vi "Fast ABR.vi"(11 "State (in)":T19) -> (3 "State (out)":T19)   [LabVIEW 2020]
uses:
  epl-vi-lib/Utility VIs/Buttons/KCheckmarkBoolean 2.ctl
  CFTS SubVIs/CFTS-Experiment State.ctl
  Typedefs/FABR-Analysis State.ctl
  <vilib>/printing/EasyPrintingControls.llb/layout_options.ctl
  <vilib>/printing/EasyPrintingControls.llb/orientation.ctl
  <vilib>/printing/EasyPrintingControls.llb/panel_scaling_for_page.ctl
  <vilib>/printing/EasyPrintingControls.llb/margins.ctl
  <vilib>/printing/EasyPrintingControls.llb/margin_values.ctl
  <vilib>/printing/EasyPrintingControls.llb/measurement_system.ctl
  <vilib>/printing/EasyPrintingControls.llb/printer_options.ctl
  <vilib>/printing/EasyPrintingControls.llb/printing_method.ctl
  <vilib>/printing/EasyPrintingControls.llb/color_or_monochrome.ctl
  <vilib>/printing/EasyPrintingControls.llb/page_header_options.ctl
  <vilib>/printing/EasyPrintingControls.llb/page_headers.ctl
  <vilib>/printing/EasyPrintingControls.llb/page_header_content_options.ctl
  Typedefs/FABR-Parameters/FABR-Parameters.xctl
  Typedefs/FABR-Status.ctl
  Typedefs/FABR-Queue Data.ctl
  Typedefs/FABR-Parameters.ctl
  Typedefs/FABR-Stimulus.ctl
  Typedefs/FABR-Sequence.ctl
  Typedefs/FABR-Order.ctl
  Typedefs/FABR-Response.ctl
  Threshold Estimation VIs/ABR3-Threshold Estimation Parameters.ctl
  Typedefs/FABR-Stimulus Condition.ctl
  epl-vi-lib/PXI DAQ VIs/AIDI/Typedefs/AIDI-Action.ctl
  CFTS SubVIs/CFTS-Options.ctl
  <vilib>/printing/EasyPrintingControls.llb/contents.ctl
  931a586e-3910-4d06-be6a-8dff1fbf7332.vi
  epl-vi-lib/Utility VIs/Math VIs/LinSpace (start-stop-step).vi
  epl-vi-lib/Utility VIs/File IO VIs/Read Write Anything/Read Anything.vi
  <vilib>/printing/EasyPrinting.llb/Easy Print VI Panel or Documentation (refnum).vi
  <vilib>/Utility/NIReport.llb/NI_ReportGenerationCore.lvlib
panel:
  in  "Params":T5(xcontrol)
  in  "Start":bool
  in  "Run":i32
  in  "Number":i32
  in  "ID":string
  in  "Stop":bool
  in  "layout options":T6={"orientation (unchanged)"=0, "panel scaling for page (unchanged)"=0, "margins"={"override VI margins (false)"=FALSE, "margins (1.00)"={"top"=1.0, "left"=1.0, "right"=1.0, "bottom"=1.0}, "measurement system (default)"=0}, "printer options"={"destination printer name (current)"="", "printing method (unchanged)"=0, "color or monochrome (unchanged)"=0}, "page header options"={"page headers (unchanged)"=0, "page header content options"={"Include VI Name"=TRUE, "Include VI Path"=TRUE, "Include Last Modification Date"=TRUE, "Include Date Printed"=TRUE, "Include Page Number"=TRUE, "Include VI Icon"=TRUE}}} {"page header options"."page headers (unchanged)" items=["Unchanged", "Include page headers", "Do not include page headers"]; "printer options"."color or monochrome (unchanged)" items=["Unchanged", "Color/grayscale", "Monochrome"]; "printer options"."printing method (unchanged)" items=["Unchanged", "Standard", "PostScript", "Bitmap"]; "panel scaling for page (unchanged)" items=["Unchanged", "No Scaling", "Scale front panel to fit"]; "orientation (unchanged)" items=["Unchanged", "portrait", "landscape"]; "margins"."measurement system (default)" items=["Default", "US", "Metric"]; "margins"."margins (1.00)"."right" format="%.2f"; "margins"."margins (1.00)"."bottom" format="%.2f"; "margins"."margins (1.00)"."top" format="%.2f"; "margins"."margins (1.00)"."left" format="%.2f"}
  in  "NOTES":string
  in  "Scale":dbl=1.0 min=1.0 max=5.0 step=0.5
  out "Frej":dbl(slide) scale=0.0..1.0
  in  "RejThr":dbl caption="Reject at (uV)"
  in  "Override":bool
  in  "AvsF Axis":dbl(slide) caption="Frequency (kHz)" min=0.0 scale=0.0..3.0 scale format="%#.2g"
  out "Raw":dbl[](graph)
  out "AvsFLegend":i32(listbox)
  out "AvsF":cluster{dbl[], dbl[]}[](graph)
  out "IOLegend":i32(listbox)
  in  "YAxis":dbl(slide) caption="Level (dB SPL)" scale=0.0..13.5
  in  "XAxis":dbl(slide) caption="Frequency (kHz)" min=0.0 scale=0.0..4.0 scale format="%#.2g"
  out "Neural":cluster{dbl[], dbl[]}[](graph)
  out "Analysis":T18
  out "finished":errorcluster
  in  "Normalize traces":T20=TRUE caption="Normalize individual traces"
  out "I-O":cluster{dbl[], dbl[]}[](graph)
  # "Freq X Level X Time"
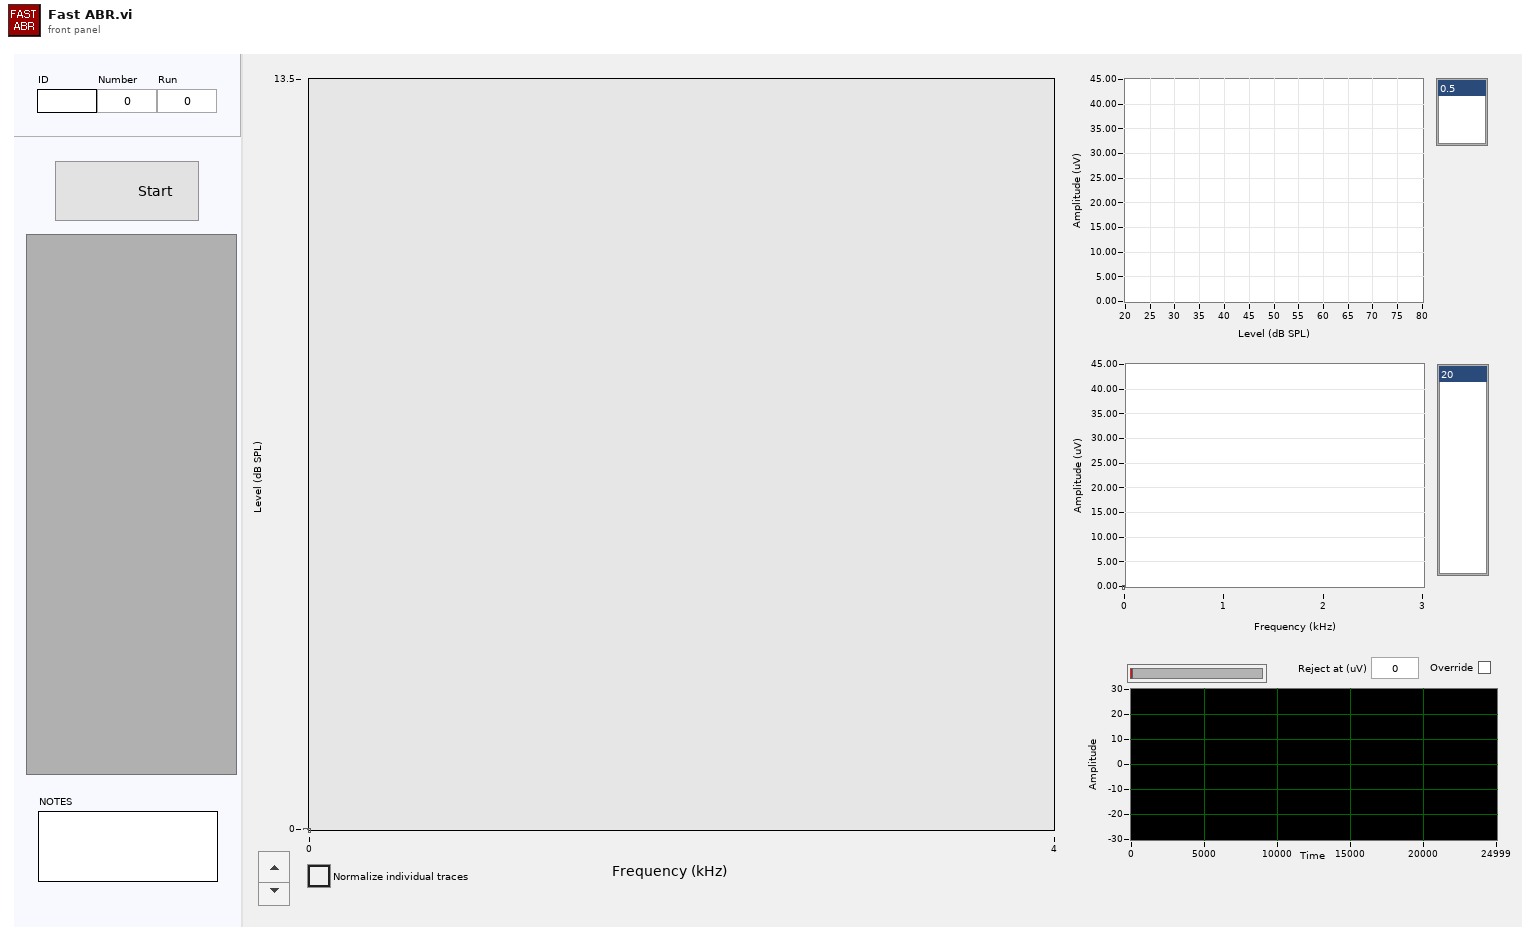
[diagram p1: front panel]
types:
  T1 = typedef "FABR-Stimulus.ctl" = cluster{"Destination":string, "Rep rate (/sec)":dbl, "Alternate Polarity":bool, "Duration (ms)":dbl, "Ramp (ms)":dbl, "Fs (Hz)":dbl, "Frame size (s)":dbl}
  T2 = typedef "FABR-Sequence.ctl" = cluster{"Freq":cluster{"Start (kHz)":dbl, "Stop (kHz)":dbl, "Step (oct)":dbl, "Skip (oct)":dbl}, "Level":cluster{"Start (dB)":i32, "Stop (dB)":i32, "Step (dB)":i32}, "Order":T3}
  T3 = typedef "FABR-Order.ctl" = enum16{"Interleaved"}
  T4 = typedef "FABR-Response.ctl" = cluster{"Gain":dbl, "Averages":i32, "Window (ms)":sgl, "Fs (Hz)":dbl, "Save raw":bool}
  T5 = cluster{"Stimulus":T1, "Sequence":T2, "Response":T4, "Reject":dbl}
  T6 = typedef "NI_ReportGenerationCore.lvlib/layout_options.ctl" = cluster{"orientation (unchanged)":T7, "panel scaling for page (unchanged)":T8, "margins":T9, "printer options":T12, "page header options":T15}
  T7 = typedef "NI_ReportGenerationCore.lvlib/orientation.ctl" = u16
  T8 = typedef "NI_ReportGenerationCore.lvlib/panel_scaling_for_page.ctl" = u16
  T9 = typedef "NI_ReportGenerationCore.lvlib/margins.ctl" = cluster{"override VI margins (false)":bool, "margins (1.00)":T10, "measurement system (default)":T11}
  T10 = typedef "NI_ReportGenerationCore.lvlib/margin_values.ctl" = cluster{"top":dbl, "left":dbl, "right":dbl, "bottom":dbl}
  T11 = typedef "NI_ReportGenerationCore.lvlib/measurement_system.ctl" = u16
  T12 = typedef "NI_ReportGenerationCore.lvlib/printer_options.ctl" = cluster{"destination printer name (current)":string, "printing method (unchanged)":T13, "color or monochrome (unchanged)":T14}
  T13 = typedef "NI_ReportGenerationCore.lvlib/printing_method.ctl" = u16
  T14 = typedef "NI_ReportGenerationCore.lvlib/color_or_monochrome.ctl" = u16
  T15 = typedef "NI_ReportGenerationCore.lvlib/page_header_options.ctl" = cluster{"page headers (unchanged)":T16, "page header content options":T17}
  T16 = typedef "NI_ReportGenerationCore.lvlib/page_headers.ctl" = u16
  T17 = typedef "NI_ReportGenerationCore.lvlib/page_header_content_options.ctl" = cluster{"Include VI Name":bool, "Include VI Path":bool, "Include Last Modification Date":bool, "Include Date Printed":bool, "Include Page Number":bool, "Include VI Icon":bool}
  T18 = typedef "FABR-Analysis State.ctl" = cluster{"Neural":dbl[][][], "CM":dbl[][][], "Metrics":dbl[][][], "Level":dbl[], "Avgs":i32[][], "Attempts":i32[][], "Navg":i32, "threshold":dbl[], "Freq":dbl[], "dt":dbl}
  T19 = typedef "CFTS-Experiment State.ctl" = cluster{"Experimenter":string, "Number":u32, "Right":string, "Left":string, "Data Folder":path, "Version":string, "End Exposure Time":dbl, "Exposure Duration":string, "Run #":cluster{"CAP":i32, "ABR":i32, "DP":i32, "VsEP":i32, "SFOAE":i32}}
  T20 = typedef "KCheckmarkBoolean 2.ctl" = bool
  T21 = typedef "FABR-Queue Data.ctl" = cluster{"Action":string, "Path":path, "Params":T22, "Threshold":T23}
  T22 = typedef "FABR-Parameters.ctl" = cluster{"Stimulus":T1, "Sequence":T2, "Response":T4, "Reject":dbl}
  T23 = typedef "ABR3-Threshold Estimation Parameters.ctl" = cluster{"Tmin (ms)":dbl, "Tmax (ms)":dbl, "CC criterion":dbl, "adjR2 criterion":dbl}
  T24 = typedef "FABR-Status.ctl" = cluster{"Freq":dbl[], "Level":dbl[], "running":bool}
  T25 = cluster{"Neural":refnum<vi>, "I-O":refnum<vi>, "AvsF":refnum<vi>}
  T26 = enum8{"Enabled", "Disabled", "Disabled and Grayed Out"}
  T27 = typedef "CFTS-Options.ctl" = cluster{"Rig ID":string, "Acoustic System IDs":cluster{"Right":string, "Left":string}, "Extension":string, "Advanced users":string[], "All advanced":bool, "Run vitals":bool, "hash":string, "Allow nonEPL":bool, "NonEPL":string[]}
  T28 = cluster{string, "appended path":path, "Params":T22, "Threshold Estimation":T23}
  T29 = typedef "NI_ReportGenerationCore.lvlib/contents.ctl" = u16
  T30 = typedef "LVPoint32TypeDef.ctl" = cluster{"Horizontal":i32, "Vertical":i32}
  T31 = typedef "ABR3-Threshold Estimation Work.ctl" = cluster{"Threshold":dbl, "Criterion":dbl, "graphs":cluster{"X":dbl[], "Y":dbl[]}[], "Power2":string, "Sigmoid":string, "Result":T32}
  T32 = typedef "ABR3-Threshold Estimation Result.ctl" = enum16{"None", "Power", "Sigmoid", "Power (noisy)", "Suprathreshold", "Invalid"}
  T33 = typedef "FABR-Stimulus Condition.ctl" = cluster{"Freq":dbl, "Findex":i32, "Level":dbl, "Lindex":i32, "Atten":dbl, "Pol":cluster{"stim":i32, "need":i32}, "Sum1":dbl[], "Sum2":dbl[], "Nacq":i32, "Natt":i32, "finished":bool}
  T34 = typedef "AIDI-Action.ctl" = enum16{"Configure", "Initialize", "Start", "Read", "Clean up", "Init & Start", "Config & Test", "Position", "Skip"}
  T35 = typedef "FABR-Runtime Data.ctl" = cluster{"AI pts/stim":i32, "gain factor":dbl, "stims/frame":i32, "NWinPts":i32, "Navgs":i32, "Tones":dbl[][], "stims":T36[], "resps":T36[], "raw":refnum<file>}
  T36 = typedef "FABR-Stimulus Ticket.ctl" = cluster{"sclIndex":i32, "Findex":i32, "Lindex":i32, "Polarity":i32, "Atten":dbl}
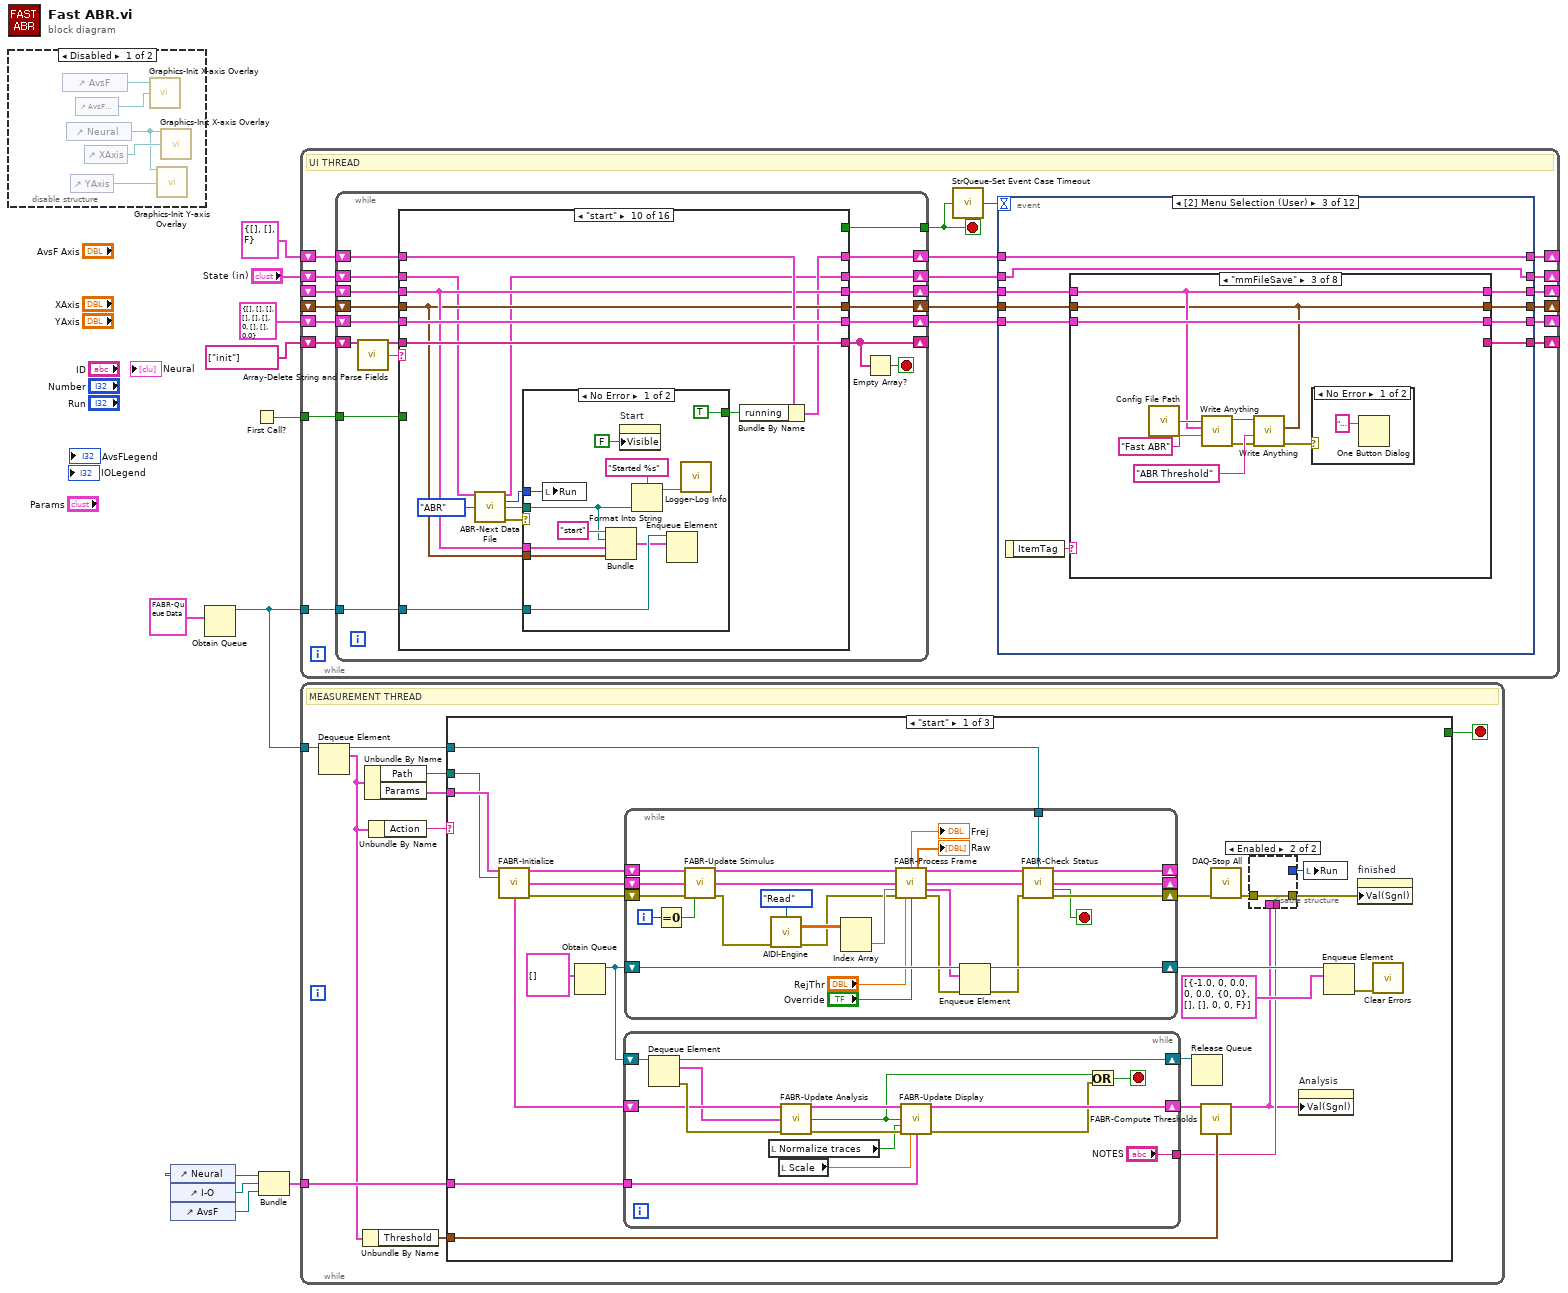
[diagram p0: block diagram]
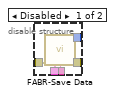
[diagram p2: hidden frame]
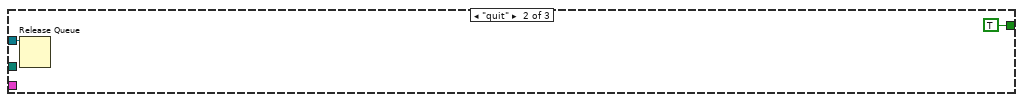
[diagram p3: hidden frame]
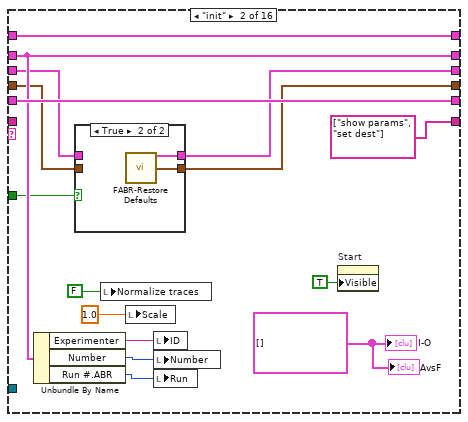
[diagram p7: hidden frame]
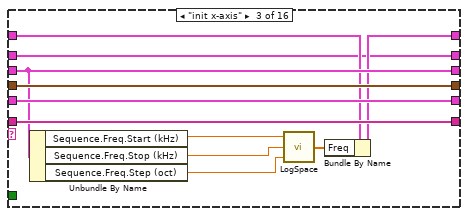
[diagram p9: hidden frame]
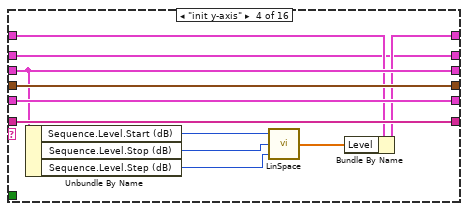
[diagram p10: hidden frame]
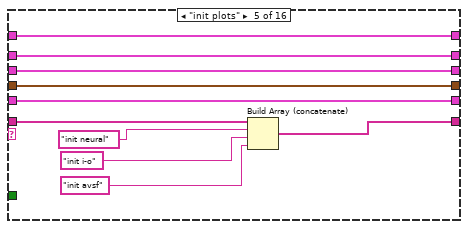
[diagram p11: hidden frame]
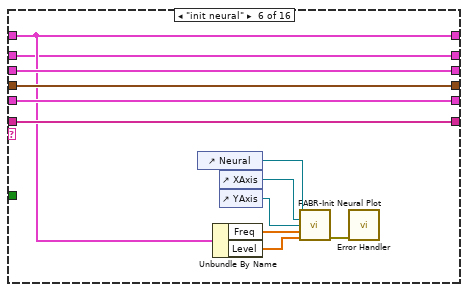
[diagram p12: hidden frame]
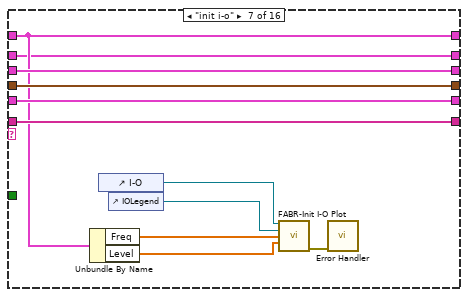
[diagram p13: hidden frame]
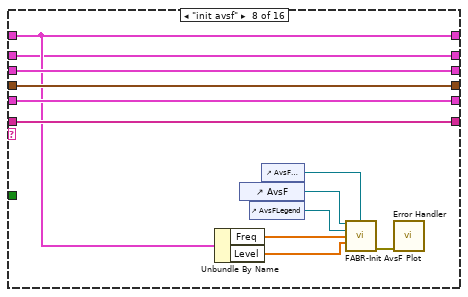
[diagram p14: hidden frame]
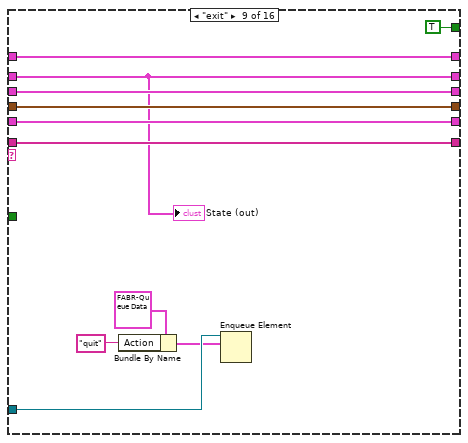
[diagram p15: hidden frame]
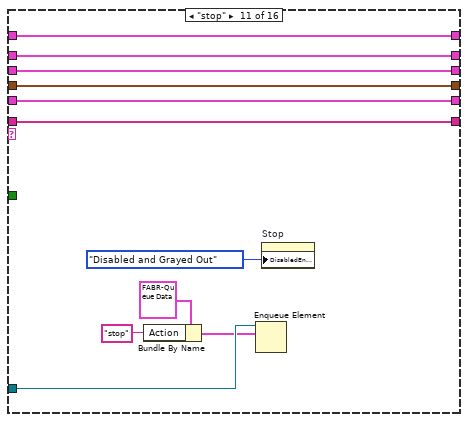
[diagram p17: hidden frame]
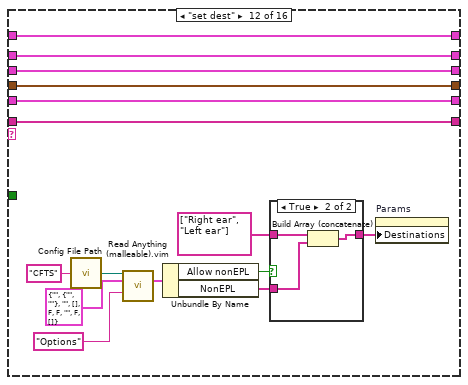
[diagram p18: hidden frame]
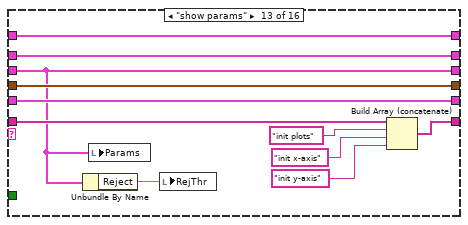
[diagram p20: hidden frame]
diagram:
  n1 = disable-structure shown="Disabled" {
    frame Disabled {
      n2 = control-ref of="AvsF"() -> (w13:refnum<vi>)
      n3 = control-ref of="Neural"() -> (w14:refnum<vi>)
      n4 = control-ref of="YAxis"() -> (w15:refnum<vi>)
      n5 = control-ref of="AvsF Axis"() -> (w12:refnum<vi>)
      n6 = control-ref of="XAxis"() -> (w16:refnum<vi>)
      n7 = call "Graphics-Init X-axis Overlay.vi"("Ctl Refnum"=w13, "X-axis slider"=w12) -> ()  [unwired: 13 in, 1 out]
      n8 = call "Graphics-Init Y-axis Overlay.vi"("Ctl Refnum"=w14, "Y-axis slider"=w15) -> ()  [unwired: 13 in, 1 out]
      n9 = call "Graphics-Init X-axis Overlay.vi"("Ctl Refnum"=w14, "X-axis slider"=w16) -> ()  [unwired: 13 in, 1 out]
    }
    frame Enabled {
    }
  }
  n10 = control-ref of="Neural"() -> (w8:refnum<vi>)
  n11 = control-ref of="I-O"() -> (w7:refnum<vi>)
  n12 = control-ref of="AvsF"() -> (w6:refnum<vi>)
  n13 = Obtain Queue(element data type=T21 {"Action"="", "Path"=path "", "Params"={"Stimulus"={"Destination"="", "Rep rate (/sec)"=0.0, "Alternate Polarity"=FALSE, "Duration (ms)"=0.0, "Ramp (ms)"=0.0, "Fs (Hz)"=0.0, "Frame size (s)"=0.0}, "Sequence"={"Freq"={"Start (kHz)"=20.0, "Stop (kHz)"=80.0, "Step (oct)"=5.0, "Skip (oct)"=0.0}, "Level"={"Start (dB)"=20, "Stop (dB)"=80, "Step (dB)"=5}, "Order"=enum."Interleaved"}, "Response"={"Gain"=0.0, "Averages"=0, "Window (ms)"=0.0, "Fs (Hz)"=25000.0, "Save raw"=FALSE}, "Reject"=0.0}, "Threshold"={"Tmin (ms)"=0.0, "Tmax (ms)"=0.0, "CC criterion"=0.0, "adjR2 criterion"=0.0}} ("output cluster")) -> (queue out=w11:refnum<queue>)  [unwired: 4 in, 2 out]
  n14 = First Call?() -> (First Call?: T/F=w3:bool)
  n15 = Bundle("Neural"=w8, "I-O"=w7, "AvsF"=w6) -> (w2:T25)  [unwired: 1 in]
  n16 = while {
    tunnel: w11 -> [w37]
    shift-right: [w25] -> _
    shift-left: _ -> [w35]
    shift-right: [w19] -> _
    shift-left: T18 {"Neural"=[], "CM"=[], "Metrics"=[], "Level"=[], "Avgs"=[], "Attempts"=[], "Navg"=0, "threshold"=[], "Freq"=[], "dt"=0.0} ("Analysis") -> [w36]
    shift-right: [w26] -> _
    shift-left: _ -> [w34]
    shift-right: [w27] -> _
    shift-left: T24 {"Freq"=[], "Level"=[], "running"=FALSE} ("Status") -> [w33]
    shift-right: [w24] -> _
    shift-left: string[] ["init"] -> [w32]
    tunnel: w3 -> [w20]
    shift-right: [w18] -> _
    shift-left: "State (in)" -> [w21]
    stop <- w23 stop-if-true
    # "UI THREAD"
    n17 = while {
      tunnel: w37 -> [w49]
      shift-right: [w46] -> _
      shift-left: w32 -> [w43]
      tunnel: [w48] -> w23
      shift-right: [w44] -> w31
      shift-left: w33 -> [w45]
      tunnel: w20 -> [w39]
      shift-right: [w50] -> w28
      shift-left: w36 -> [w53]
      shift-right: [w52] -> w30
      shift-left: w34 -> [w55]
      shift-right: [w51] -> w29
      shift-left: w35 -> [w54]
      shift-right: [w38] -> w17
      shift-left: w21 -> [w40]
      stop <- w47 stop-if-true
      n18 = call "Array-Delete String and Parse Fields.vi"("Array in"=w43) -> ("Array out"=w42:string[], "Field 1"=w41:string)  [unwired: 10 in, 3 out]
      n19 = case shown="\"start\"" w41 {
        tunnel: w55 -> [w61 w62 w92 w103 w113 w125 w136 w148 w154 w169 w191 w210 w225 w232 w259 w273]
        tunnel: w54 -> [w60 w63 w89 w100 w112 w124 w135 w147 w155 w170 w192 w209 w215 w230 w258 w272]
        tunnel: w53 -> [w59 w77 w91 w102 w111 w123 w134 w146 w159 w173 w195 w208 w224 w226 w255 w268]
        tunnel: [w61 w65 w92 w103 w113 w125 w136 w148 w154 w169 w191 w210 w225 w232 w259 w273] -> w52
        tunnel: [w60 w64 w89 w100 w112 w124 w135 w147 w155 w170 w192 w209 w215 w230 w258 w272] -> w51
        tunnel: [w59 w77 w91 w102 w111 w123 w134 w146 w159 w173 w195 w208 w224 w231 w255 w268] -> w50
        tunnel: w49 -> [_ _ _ _ _ _ _ _ w153 w168 w190 _ _ _ _ _]
        tunnel: [w58 string[] ["show params", "set dest"] w90 w101 w108 w122 w133 w145 w158 w172 w194 w207 w222 w235 w257 w270] -> w46
        tunnel: w42 -> [w58 _ w90 w101 w110 w122 w133 w145 w158 w172 w194 w207 w223 _ w257 w270]
        tunnel: [_ _ _ _ _ _ _ _ TRUE _ _ _ _ _ _ _] -> w48
        tunnel: w45 -> [w57 w76 w85 w96 w109 w121 w129 w141 w156 w171 w193 w206 w218 w234 w256 w266]
        tunnel: [w57 w76 w84 w95 w109 w121 w129 w141 w156 w167 w193 w206 w218 w233 w256 w266] -> w44
        tunnel: w40 -> [w56 w72 w82 w93 w104 w114 w126 w137 w152 w166 w188 w205 w216 w238 w254 w265]
        tunnel: w39 -> [_ w66 _ _ _ _ _ _ _ _ _ _ _ _ _ _]
        tunnel: [w56 w72 w82 w93 w104 w114 w126 w137 w152 w165 w188 w205 w216 w238 w254 w265] -> w38
        frame Default {
        }
        frame "init" {
          w67 = cluster{dbl[], dbl[]}[] [] ("XY Graph")
          n20 = Unbundle By Name(w72) -> ("Experimenter"=w73:string, "Number"=w74:u32, "Run #.ABR"=w75:i32)
          n21 = case shown="True" w66 {
            tunnel: w62 -> [w79 _]
            tunnel: [w79 w80] -> w65
            tunnel: [w78 w81] -> w64
            tunnel: w63 -> [w78 _]
            frame False {
            }
            frame True {
              n22 = call "FABR-Restore Defaults.vi"() -> ("Params"=w81:T22, "Threshold Estimation"=w80:T23)  [unwired: 13 in, 1 out]
            }
          }
          n23 = local write "Normalize traces"(T20 FALSE ("Normalize traces")) -> ()
          n24 = local write "Scale"(1.0 ("Scalebar")) -> ()
          n25 = local write "ID"(w73) -> ()
          n26 = local write "Number"(w74) -> ()
          n27 = local write "Run"(w75) -> ()
          n28 = property on="Start" class="Bool"("Visible"=TRUE) -> ()  [unwired: 2 in, 2 out]
          "I-O" <- w67
          "AvsF" <- w67
        }
        frame "init x-axis" {
          n29 = Unbundle By Name(w89) -> ("Sequence.Freq.Start (kHz)"=w88:dbl, "Sequence.Freq.Stop (kHz)"=w87:dbl, "Sequence.Freq.Step (oct)"=w86:dbl)
          n30 = call "LogSpace.vi"("Start"=w88, "Stop"=w87, "Step"=w86) -> ("Array"=w83:dbl[])  [unwired: 3 in, 1 out]
          n31 = Bundle By Name(cluster=w85, "Freq"=w83) -> (w84:T24)
        }
        frame "init y-axis" {
          n32 = Unbundle By Name(w100) -> ("Sequence.Level.Start (dB)"=w99:i32, "Sequence.Level.Stop (dB)"=w98:i32, "Sequence.Level.Step (dB)"=w97:i32)
          n33 = call-poly "LinSpace.vi"("Step"=w97, "Stop"=w98, "Start"=w99) -> ("Array"=w94:dbl[])  [unwired: 1 in, 1 out]
          n34 = Bundle By Name(cluster=w96, "Level"=w94) -> (w95:T24)
        }
        frame "init plots" {
          n35 = Build Array (concatenate)(w110, "init neural", "init i-o", "init avsf") -> (w108:string[])
        }
        frame "init neural" {
          n36 = control-ref of="Neural"() -> (w120:refnum<vi>)
          n37 = Unbundle By Name(w121) -> ("Freq"=w116:dbl[], "Level"=w115:dbl[])
          n38 = control-ref of="XAxis"() -> (w118:refnum<vi>)
          n39 = control-ref of="YAxis"() -> (w117:refnum<vi>)
          n40 = call "FABR-Init Neural Plot.vi"("XYGraph in"=w120, "XAxis"=w118, "YAxis"=w117, "Freq"=w116, "Level"=w115) -> ("error out"=w119:errorcluster)  [unwired: 10 in]
          n41 = call "Error Handler.vi"("error in (no error)"=w119) -> ()  [unwired: 12 in, 3 out]
        }
        frame "init i-o" {
          n42 = Unbundle By Name(w129) -> ("Freq"=w128:dbl[], "Level"=w127:dbl[])
          n43 = control-ref of="I-O"() -> (w131:refnum<vi>)
          n44 = control-ref of="IOLegend"() -> (w132:refnum<vi>)
          n45 = call "FABR-Init I-O Plot.vi"("I-O"=w131, "IOLegend"=w132, "Freq"=w128, "Level"=w127) -> ("error out"=w130:errorcluster)  [unwired: 11 in]
          n46 = call "Error Handler.vi"("error in (no error)"=w130) -> ()  [unwired: 12 in, 3 out]
        }
        frame "init avsf" {
          n47 = Unbundle By Name(w141) -> ("Freq"=w140:dbl[], "Level"=w139:dbl[])
          n48 = control-ref of="AvsF"() -> (w142:refnum<vi>)
          n49 = control-ref of="AvsFLegend"() -> (w143:refnum<vi>)
          n50 = control-ref of="AvsF Axis"() -> (w144:refnum<vi>)
          n51 = call "FABR-Init AvsF Plot.vi"("Graph"=w142, "FreqAxisLabel"=w144, "Legend"=w143, "Freq"=w140, "Level"=w139) -> ("error out"=w138:errorcluster)  [unwired: 10 in]
          n52 = call "Error Handler.vi"("error in (no error)"=w138) -> ()  [unwired: 12 in, 3 out]
        }
        frame "exit" {
          n53 = Bundle By Name(cluster=T21 {"Action"="", "Path"=path "", "Params"={"Stimulus"={"Destination"="", "Rep rate (/sec)"=0.0, "Alternate Polarity"=FALSE, "Duration (ms)"=0.0, "Ramp (ms)"=0.0, "Fs (Hz)"=0.0, "Frame size (s)"=0.0}, "Sequence"={"Freq"={"Start (kHz)"=20.0, "Stop (kHz)"=80.0, "Step (oct)"=5.0, "Skip (oct)"=0.0}, "Level"={"Start (dB)"=20, "Stop (dB)"=80, "Step (dB)"=5}, "Order"=enum."Interleaved"}, "Response"={"Gain"=0.0, "Averages"=0, "Window (ms)"=0.0, "Fs (Hz)"=25000.0, "Save raw"=FALSE}, "Reject"=0.0}, "Threshold"={"Tmin (ms)"=0.0, "Tmax (ms)"=0.0, "CC criterion"=0.0, "adjR2 criterion"=0.0}} ("output cluster"), "Action"="quit") -> (w150:T21)
          n54 = Enqueue Element(queue=w153, element=w150) -> ()  [unwired: 2 in, 3 out]
          "State (out)" <- w152
        }
        frame "start" {
          n55 = call "ABR-Next Data File.vi"("State in"=w166, "CAP or ABR"=enum16{"CAP", "ABR"}."ABR") -> ("State out"=w165:T19, "Run"=w162:i32, "appended path"=w164:path, "error out"=w163:errorcluster)  [unwired: 10 in]
          n56 = case shown="No Error" w163 {
            tunnel: w170 -> [w184 _]
            tunnel: w169 -> [w183 _]
            tunnel: w168 -> [w182 _]
            tunnel: w164 -> [w176 _]
            tunnel: w162 -> [w179 _]
            tunnel: [TRUE ("running") _] -> w161
            frame No Error {
              n57 = local write "Run"(w179) -> ()
              n58 = Bundle("start", "appended path"=w176, "Params"=w184, "Threshold Estimation"=w183) -> (w174:T28)  [unwired: 1 in]
              n59 = property on="Start" class="Bool"("Visible"=FALSE) -> ()  [unwired: 2 in, 2 out]
              n60 = Format Into String(format string="Started %s", w176) -> (resulting string=w177:string)  [unwired: 2 in, 1 out]
              n61 = Enqueue Element(queue=w182, element=w174) -> ()  [unwired: 2 in, 3 out]
              n62 = call "Logger-Log Info.vi"("Message"=w177) -> ()  [unwired: 14 in, 1 out]
            }
            frame Error {
            }
          }
          n63 = Bundle By Name(cluster=w171, "running"=w161) -> (w167:T24)
        }
        frame "stop" {
          n64 = Bundle By Name(cluster=T21 {"Action"="", "Path"=path "", "Params"={"Stimulus"={"Destination"="", "Rep rate (/sec)"=0.0, "Alternate Polarity"=FALSE, "Duration (ms)"=0.0, "Ramp (ms)"=0.0, "Fs (Hz)"=0.0, "Frame size (s)"=0.0}, "Sequence"={"Freq"={"Start (kHz)"=20.0, "Stop (kHz)"=80.0, "Step (oct)"=5.0, "Skip (oct)"=0.0}, "Level"={"Start (dB)"=20, "Stop (dB)"=80, "Step (dB)"=5}, "Order"=enum."Interleaved"}, "Response"={"Gain"=0.0, "Averages"=0, "Window (ms)"=0.0, "Fs (Hz)"=25000.0, "Save raw"=FALSE}, "Reject"=0.0}, "Threshold"={"Tmin (ms)"=0.0, "Tmax (ms)"=0.0, "CC criterion"=0.0, "adjR2 criterion"=0.0}} ("output cluster"), "Action"="stop") -> (w185:T21)
          n65 = Enqueue Element(queue=w190, element=w185) -> ()  [unwired: 2 in, 3 out]
          n66 = property on="Stop" class="Bool"("DisabledEnum"=T26."Disabled and Grayed Out" ("Disabled")) -> ()  [unwired: 2 in, 2 out]
        }
        frame "set dest" {
          n67 = call "Config File Path.vi"("AppName"="CFTS") -> ("Default config file name"=w203:path)
          n68 = call "Read Anything (malleable).vim"("Config file path"=w203, "Options in"=T27 {"Rig ID"="", "Acoustic System IDs"={"Right"="", "Left"=""}, "Extension"="", "Advanced users"=[], "All advanced"=FALSE, "Run vitals"=FALSE, "hash"="", "Allow nonEPL"=FALSE, "NonEPL"=[]} ("Options"), "Section"="Options") -> ("Options out"=w200:T27)  [unwired: 9 in, 3 out]
          n69 = Unbundle By Name(w200) -> ("Allow nonEPL"=w197:bool, "NonEPL"=w196:string[])
          n70 = case shown="True" w197 {
            tunnel: string[] ["Right ear", "Left ear"] -> [w211 w213]
            tunnel: [w211 w212] -> w198
            tunnel: w196 -> [_ w214]
            frame False {
            }
            frame True {
              n71 = Build Array (concatenate)(w213, w214) -> (w212:string[])
            }
          }
          n72 = property on="Params" class="FABR-Parameters (strict)"("Destinations"=w198) -> ()  [unwired: 2 in, 2 out]
        }
        frame "show params" {
          n73 = Unbundle By Name(w215) -> ("Reject"=w219:dbl)
          n74 = local write "Params"(w215) -> ()
          n75 = local write "RejThr"(w219) -> ()
          n76 = Build Array (concatenate)(w223, "init plots" ("element"), "init x-axis", "init y-axis") -> (w222:string[])
        }
        frame "open" {
          n77 = Unbundle By Name(w238) -> ("Data Folder"=w236:path)
          n78 = call "FileIO-Open Dialog (multiple).vi"("Default Folder"=w236, "pattern (all files)"="*") -> ("error out"=w227:errorcluster, "cancelled"=w228:bool, "Paths"=w229:path[])  [unwired: 7 in]
          n79 = case shown="False" w228 {
            tunnel: w227 -> [w247 _]
            tunnel: w226 -> [_ w253]
            tunnel: [w245 w253] -> w231
            tunnel: w229 -> [w246 _]
            tunnel: [string[] ["plot traces", "plot metrics", "init plots"] _] -> w235
            tunnel: w234 -> [w241 w252]
            tunnel: [w240 w252] -> w233
            tunnel: w232 -> [w239 _]
            frame False {
              n80 = disable-structure shown="Disabled" {
                disable-tunnel: w247 -> [w251 _]
                disable-tunnel: w246 -> [w250 _]
                disable-tunnel: [w249 _] -> w245
                disable-tunnel: w239 -> [w248 _]
                frame Disabled {
                  n81 = call "FABR-Read Data.vi"("Data files"=w250, "Threshold Estimation"=w248, "error in (no error)"=w251) -> ("Analysis"=w249:T18)  [unwired: 11 in, 1 out]
                }
                frame Enabled {
                }
              }
              n82 = Unbundle By Name(w245) -> ("Freq"=w243:dbl[], "Level"=w242:dbl[])
              n83 = Bundle By Name(cluster=w241, "Freq"=w243, "Level"=w242) -> (w240:T24)
            }
            frame True {
            }
          }
        }
        frame "plot traces" {
          n84 = disable-structure shown="Disabled" {
            disable-tunnel: w255 -> [w261 _]
            frame Disabled {
              n85 = control-ref of="Neural"() -> (w260:refnum<vi>)
              n86 = call "FABR-Plot Traces.vi"("Analysis"=w261, "Neural Ref"=w260, "Normalize individual?"="Normalize traces", "Scale"="Scale") -> ("error out"=w262:errorcluster)  [unwired: 11 in]
              n87 = call "FABR-Plot Thresholds.vi"("Analysis"=w261, "Neural Ref"=w260, "error in (no error)"=w262) -> ()  [unwired: 12 in, 1 out]
            }
            frame Enabled {
            }
          }
          n88 = call "Error Handler.vi"() -> ()  [unwired: 13 in, 3 out]
        }
        frame "plot metrics" {
          n89 = control-ref of="I-O"() -> (w271:refnum<vi>)
          n90 = call "FABR-Plot I-O.vi"("Analysis"=w268, "I-O"=w271) -> ("error out"=w267:errorcluster)  [unwired: 13 in]
          n91 = control-ref of="AvsF"() -> (w269:refnum<vi>)
          n92 = call "FABR-Plot AvsF.vi"("Analysis"=w268, "I-O"=w269, "error in (no error)"=w267) -> ()  [unwired: 12 in, 1 out]
        }
      }
      n93 = Empty Array?(array=w46) -> (empty?=w47:bool)
    }
    n94 = call "StrQueue-Set Event Case Timeout.vi"("Quit"=w23) -> ("timeout"=w22:i32)  [unwired: 14 in]
    n95 = event shown="[2] Menu Selection (User)" {
      selector: _ -> [_ _ _ _ _ _ _ _ _ _ _ _]
      dyn-events: _ -> [_ _ _ _ _ _ _ _ _ _ _ _]
      timeout: w22 -> [_ _ _ _ _ _ _ _ _ _ _ _]
      tunnel: w29 -> [w275 w285 w294 w354 w370 w377 w381 w389 w400 w407 _ w422]
      tunnel: [w275 w285 w293 w354 w370 w374 w381 w389 w400 w407 w409 w422] -> w25
      tunnel: w28 -> [w278 w284 w292 w353 w359 w376 w383 w388 w398 w406 w415 _]
      tunnel: [w276 w282 w289 w350 w357 w375 w380 w387 w399 w405 w414 w420] -> w26
      tunnel: w30 -> [w276 w282 w290 w350 w357 w375 w380 w387 w399 w405 w414 w420]
      tunnel: [_ string[] ["exit"] w288 _ _ _ string[] ["start"] string[] ["stop"] _ w402 w413 string[] ["plot traces"]] -> w24
      tunnel: w31 -> [w277 w280 w286 w349 w369 w372 w382 w386 w396 w404 w412 w419]
      tunnel: [w277 w280 w286 w349 w369 w372 w382 w386 w395 w404 w412 w419] -> w27
      tunnel: [w278 w284 w291 w353 w359 w376 w383 w388 w398 w406 w415 w421] -> w19
      tunnel: [w274 w279 w287 w348 w355 w371 w378 w384 w392 w401 w410 w417] -> w18
      tunnel: w17 -> [w274 w279 w287 w348 w355 w371 w378 w384 w392 w401 w410 w417]
      event Timeout {
        n96 = event-data() -> ()  [unwired: 1 in, 1 out]
      }
      event Panel Close? {
        n97 = event-data() -> ()  [unwired: 1 in, 1 out]
        n98 = event-data("Discard?"=TRUE) -> ()  [unwired: 1 in, 1 out]
      }
      event Menu Selection (User) {
        n99 = event-data() -> ("ItemTag"=w295:string)  [unwired: 1 in]
        n100 = case shown="\"mmFileSave\"" w295 {
          tunnel: w294 -> [w298 w304 w319 w327 w333 w337 w339 w347]
          tunnel: [w298 w299 w319 w327 w333 w337 w338 w347] -> w293
          tunnel: w292 -> [w297 w307 w321 w326 w329 w336 w343 w345]
          tunnel: [w297 w307 w321 w326 w329 w336 w343 w345] -> w291
          tunnel: w290 -> [w296 w302 w313 w325 w328 w335 w342 w344]
          tunnel: [w296 w300 w313 w325 w328 w335 w341 w344] -> w289
          tunnel: [_ w301 _ string[] ["open"] _ string[] ["exit"] _ _] -> w288
          frame Default {
          }
          frame "mmFileRestore" {
            n101 = call "FABR-Restore Defaults.vi"() -> ("Params"=w305:T22, "Threshold Estimation"=w303:T23, "error out"=w306:errorcluster)  [unwired: 13 in]
            n102 = case shown="No Error" w306 {
              tunnel: w305 -> [w310 _]
              tunnel: w304 -> [_ w312]
              tunnel: [w310 w312] -> w299
              tunnel: w303 -> [w308 _]
              tunnel: w302 -> [_ w311]
              tunnel: [w308 w311] -> w300
              tunnel: [string[] ["show params"] _] -> w301
              frame No Error {
              }
              frame Error {
              }
            }
          }
          frame "mmFileSave" {
            n103 = call "Config File Path.vi"() -> ("Default config file name"=w320:path)  [unwired: 1 in]
            n104 = call "Write Anything.vi"("Section Name (Name of \"Anything\")"="Fast ABR" ("Section Name (Name of \"Anything\")"), "Anything"=w319, "Path (dialog)"=w320) -> ("Error Out"=w315:errorcluster, "Path out"=w316:path)  [unwired: 7 in]
            n105 = call "Write Anything.vi"("Error In"=w315, "Section Name (Name of \"Anything\")"="ABR Threshold" ("Section Name (Name of \"Anything\")"), "Anything"=w313, "Path (dialog)"=w316) -> ("Error Out"=w314:errorcluster)  [unwired: 6 in, 1 out]
            n106 = case shown="No Error" w314 {
              selector: w314 -> [_ w323]
              frame No Error {
                n107 = One Button Dialog(message="Defaults saved.") -> ()  [unwired: 1 in, 1 out]
              }
              frame Error {
                n108 = call "Error Handler.vi"("error in (no error)"=w323) -> ()  [unwired: 12 in, 3 out]
              }
            }
          }
          frame "mmFileOpen" {
          }
          frame "mmFilePrint" {
            w332 = T29 1 items=["Complete front panel", "Visible portion of front panel", "Icon, description, panel and diagram", "Documentation: Using the panel", "Documentation: Using as a subVI", "Documentation: Complete", "Documentation: Custom"] ("contents (complete front panel)")
            n109 = control-ref of="This VI"() -> (w330:refnum<vi>)
            n110 = call-poly <vilib>:"Easy Print VI Panel or Documentation.vi"("layout options"="layout options", "contents (complete front panel)"=w332, "VI reference"=w330) -> ()  [unwired: 7 in, 2 out]
          }
          frame "mmFileExit" {
          }
          frame "mmEditOptions" {
            n111 = control-ref of="This VI"() -> (w340:refnum<vi>)
            n112 = call "FABR-Options Dialog.vi"("Params In"=w339, "Parent VI"=w340, "Threshold Estimation In"=w342) -> ("Params Out"=w338:T22, "Threshold Estimation Out"=w341:T23)  [unwired: 10 in, 1 out]
          }
          frame "mmHelpManual" {
            n113 = call "CFTS-Open Help Topic.vi"("Topic Keyword"="ABR/CAP") -> ()  [unwired: 14 in, 1 out]
          }
        }
      }
      event "Neural": Shortcut Menu Activation? {
        n114 = event-data() -> ()  [unwired: 1 in, 1 out]
        n115 = Unbundle By Name(w353) -> ("Neural"=w352:dbl[][][])
        n116 = Empty Array?(array=w352) -> (empty?=w351:bool)
        n117 = event-data("Discard?"=w351) -> ()  [unwired: 1 in, 1 out]
      }
      event "Neural": Shortcut Menu Selection (User) {
        n118 = event-data() -> ("CtlRef"=w368:refnum<vi>, "Coords"=w367:T30)  [unwired: 1 in]
        n119 = invoke class="XYGraph (strict)" method="Map Coords To XY"(reference=w368, "Coords"=w367) -> ("XY"=w366:cluster{"X":dbl, "Y":dbl})  [unwired: 5 in, 6 out]
        n120 = Unbundle By Name(w359) -> ("Level"=w360:dbl[], "Neural"=w363:dbl[][][])
        n121 = Unbundle By Name(w359) -> ("dt"=w358:dbl)
        n122 = Unbundle By Name(w366) -> ("X"=w365:dbl)
        n123 = Round Toward -Infinity(1:w365) -> (0:w364:dbl)
        n124 = To Long Integer(number=w364) -> (32bit integer=w362:i32)
        n125 = Index Array(array=w363, index (dim 0)=w362) -> (element=w361:dbl[][])  [unwired: 2 in]
        n126 = call "ABR3-Estimate Threshold.vi"("Level (in)"=w360, "Neural"=w361, "dt (us)"=w358, "Threshold Estimation"=w357) -> ("Work"=w356:T31)  [unwired: 9 in, 2 out]
        n127 = call "ABR3-Show Threshold Estimation Work.vi"("work"=w356) -> ()  [unwired: 15 in]
      }
      event "RejThr": Value Change {
        n128 = event-data() -> ("NewVal"=w373:dbl)  [unwired: 1 in]
        n129 = Bundle By Name(cluster=w377, "Reject"=w373) -> (w374:T22)
      }
      event "Start": Value Change {
        n130 = event-data() -> ()  [unwired: 1 in, 1 out]
      }
      event "Stop": Value Change {
        n131 = event-data() -> ()  [unwired: 1 in, 1 out]
      }
      event "finished": Value Change {
        n132 = event-data() -> ("NewVal"=w393:errorcluster)  [unwired: 1 in]
        n133 = call "Error Handler.vi"("error in (no error)"=w393) -> ()  [unwired: 12 in, 3 out]
        n134 = Bundle By Name(cluster=w396, "running"=FALSE) -> (w395:T24)
        n135 = property on="Start" class="Bool"("Visible"=TRUE) -> ()  [unwired: 2 in, 2 out]
        n136 = call "Beeper.vi"() -> ()  [unwired: 5 in, 1 out]
        n137 = local write "NOTES"("" ("NOTES")) -> ()
        n138 = property on="Stop" class="Bool"("DisabledEnum"=T26."Enabled" ("Disabled")) -> ()  [unwired: 2 in, 2 out]
      }
      event "Scale": Value Change {
        n139 = event-data() -> ()  [unwired: 1 in, 1 out]
        n140 = Unbundle By Name(w404) -> ("running"=w403:bool)
        n141 = case shown="False" w403 {
          tunnel: [string[] ["plot traces"] _] -> w402
          frame False {
          }
          frame True {
          }
        }
      }
      event "Params": Value Change {
        n142 = event-data() -> ("NewVal"=w409:T5)  [unwired: 1 in]
        n143 = Unbundle By Name(w412) -> ("running"=w411:bool)
        n144 = case shown="False" w411 {
          tunnel: [string[] ["init plots", "init x-axis", "init y-axis"] _] -> w413
          frame False {
          }
          frame True {
          }
        }
      }
      event Value Change {
        n145 = event-data() -> ("NewVal"=w421:T18)  [unwired: 1 in]
      }
    }
  }
  n146 = while {
    tunnel: w11 -> [w430]
    tunnel: w2 -> [w431]
    stop <- w429 stop-if-true
    # "MEASUREMENT THREAD"
    n147 = Dequeue Element(queue=w430) -> (queue out=w428:refnum<queue>, element=w424:T21)  [unwired: 2 in, 2 out]
    n148 = Unbundle By Name(w424) -> ("Threshold"=w423:T23)
    n149 = Unbundle By Name(w424) -> ("Path"=w425:path, "Params"=w426:T22)
    n150 = Unbundle By Name(w424) -> ("Action"=w427:string)
    n151 = case shown="\"start\"" w427 {
      tunnel: w431 -> [w453 _ _]
      tunnel: [_ TRUE _] -> w429
      tunnel: w428 -> [w432 w503 _]
      tunnel: w426 -> [w447 _ _]
      tunnel: w425 -> [w444 _ _]
      tunnel: w423 -> [w445 _ _]
      frame "start" {
        n152 = call "FABR-Initialize.vi"("Params"=w447, "Path"=w444) -> ("Runtime"=w451:T35, "SCL"=w443:cluster{T33[]}[], "Analysis"=w448:T18, "error out"=w452:errorcluster)  [unwired: 10 in]
        n153 = Obtain Queue(element data type=T33[] [] ("Array")) -> (queue out=w441:refnum<queue>)  [unwired: 4 in, 2 out]
        n154 = while {
          shift-right: [w473] -> w438
          shift-left: w441 -> [w474]
          shift-right: [w467] -> w434
          shift-left: w448 -> [w469]
          tunnel: ["NOTES"] -> w437
          tunnel: w453 -> [w462]
          stop <- w471 stop-if-true
          n155 = Dequeue Element(queue=w474) -> (queue out=w473:refnum<queue>, element=w468:T33[], error out=w472:errorcluster)  [unwired: 2 in, 1 out]
          n156 = local read "Normalize traces"() -> (w464:T20)
          n157 = local read "Scale"() -> (w460:dbl)
          n158 = call "FABR-Update Analysis.vi"("Analysis in"=w469, "update"=w468, "error in (no error)"=w472) -> ("Analysis out"=w463:T18, "finished"=w461:bool, "error out"=w466:errorcluster)  [unwired: 10 in]
          n159 = call "FABR-Update Display.vi"("Analysis in"=w463, "finished"=w461, "Normalize traces"=w464, "error in (no error)"=w466, "scale"=w460, "Cluster"=w462) -> ("Analysis thru"=w467:T18, "error out"=w465:errorcluster)  [unwired: 8 in]
          n160 = Or(x=w461, y=w465) -> (x .or. y?=w471:bool)
        }
        n161 = while {
          shift-right: [w498] -> w442
          shift-left: w452 -> [w499]
          shift-right: [w495] -> _
          shift-left: w451 -> [w502]
          shift-right: [w477] -> _
          shift-left: w443 -> [w500]
          shift-right: [w496] -> w440
          shift-left: w441 -> [w497]
          tunnel: w432 -> [w478]
          i -> [w494]
          stop <- w479 stop-if-true
          # "stepsize"
          # "max SPL"
          # "array of levels"
          # "current SPL"
          n162 = Equal To 0?(x=w494) -> (x = 0?=w493:bool)
          n163 = call "FABR-Update Stimulus.vi"("Runtime in"=w502, "SCL in"=w500, "error in (no error)"=w499, "start"=w493) -> ("Runtime out"=w501:T35, "SCL thru"=w476:cluster{T33[]}[], "error out"=w488:errorcluster)  [unwired: 9 in]
          n164 = call "AIDI-Engine.vi"("Action"=AIDI-Action."Read", "error in (no error)"=w488) -> ("AI"=w487:dbl[][], "error out"=w486:errorcluster)  [unwired: 8 in, 4 out]
          n165 = Index Array(array=w487) -> (element=w492:dbl[])  [unwired: 2 in]
          n166 = call "FABR-Process Frame.vi"("Runtime in"=w501, "SCL in"=w476, "AI Waveforms"=w492, "error in (no error)"=w486, "Reject"="RejThr", "override"="Override") -> ("reject fraction"=→"Frej":dbl, "Raw"=→"Raw":dbl[], "Runtime out"=w484:T35, "SCL out"=w475:cluster{T33[]}[], "update"=w482:T33[], "error out"=w485:errorcluster)  [unwired: 4 in]
          n167 = Enqueue Element(queue=w497, element=w482, error in (no error)=w485) -> (queue out=w496:refnum<queue>, error out=w483:errorcluster)  [unwired: 1 in, 1 out]
          n168 = call "FABR-Check Status.vi"("Runtime in"=w484, "queue"=w478, "SCL in"=w475, "error in (no error)"=w483) -> ("Runtime thru"=w495:T35, "SCL thru"=w477:cluster{T33[]}[], "finished"=w479:bool, "error out"=w498:errorcluster)  [unwired: 8 in]
        }
        n169 = Release Queue(queue=w438) -> ()  [unwired: 2 in, 3 out]
        n170 = call "FABR-Compute Thresholds.vi"("Analysis in"=w434, "Threshold Estimation"=w445) -> ("Analysis out"=w435:T18)  [unwired: 13 in]
        n171 = call "DAQ-Stop All.vi"("error in (no error)"=w442) -> ("error out"=w433:errorcluster)  [unwired: 14 in]
        n172 = disable-structure shown="Enabled" {
          disable-tunnel: [w458 w459] -> w450
          disable-tunnel: w437 -> [w457 _]
          disable-tunnel: [w456 _] -> w436
          disable-tunnel: w435 -> [w455 _]
          disable-tunnel: w433 -> [w454 w459]
          frame Disabled {
            n173 = call "FABR-Save Data.vi"("error in (no error)"=w454, "Analysis"=w455, "Notes"=w457) -> ("Run #"=w456:i16, "error out"=w458:errorcluster)  [unwired: 9 in, 2 out]
          }
          frame Enabled {
          }
        }
        n174 = property on="Analysis" class="Clust (strict)"("Val(Sgnl)"=w435) -> ()  [unwired: 2 in, 2 out]
        n175 = local write "Run"(w436) -> ()
        n176 = Enqueue Element(queue=w440, element=T33[] [{"Freq"=-1.0, "Findex"=0, "Level"=0.0, "Lindex"=0, "Atten"=0.0, "Pol"={"stim"=0, "need"=0}, "Sum1"=[], "Sum2"=[], "Nacq"=0, "Natt"=0, "finished"=FALSE}]) -> (error out=w449:errorcluster)  [unwired: 2 in, 2 out]
        n177 = property on="finished" class="Clust (strict)"("Val(Sgnl)"=w450) -> ()  [unwired: 2 in, 2 out]
        n178 = call <vilib>:"Clear Errors.vi"("error in (no error)"=w449) -> ()  [unwired: 5 in, 2 out]
      }
      frame "quit" {
        n179 = Release Queue(queue=w503) -> ()  [unwired: 2 in, 3 out]
      }
      frame Default {
      }
    }
  }
